vi "Set Scrollbars.vi"(8 "error in (no error)":errorcluster, 10 "Scrollbars":bool, 11 "2DArrayManager in":refnum<class "2DArrayManager.lvclass">) -> (0 "error out":errorcluster, 3 "2DArrayManager out":refnum<class "2DArrayManager.lvclass">)   [LabVIEW 2020, in "OOPanel.lvlib" / "2DArrayManager.lvclass"]
uses:
  2DArrayManager.lvclass
  2DArrayManager.lvclass/2DArrayManager.ctl
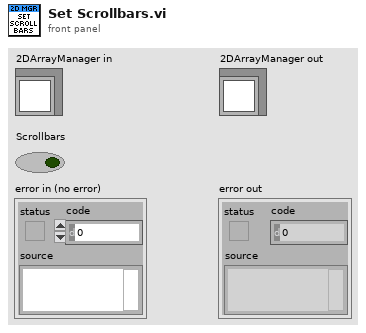
[diagram p1: front panel]
types:
  T1 = typedef "OOPanel.lvlib/2DArrayManager.lvclass/Options.ctl" = cluster{"Running":bool, "Borders":bool, "Background":u32, "V Scroll":bool, "H Scroll":bool, "Blank":refnum<class "2DPanelBlank.lvclass">}
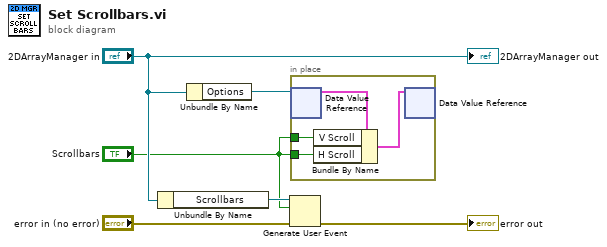
[diagram p0: block diagram]
diagram:
  n1 = Unbundle By Name("2DArrayManager in") -> ("Scrollbars"=w6:refnum<user-event>)
  n2 = Unbundle By Name("2DArrayManager in") -> ("Options"=w3:refnum<data-value>)
  n3 = Generate User Event(user event=w6, event data cluster="Scrollbars", error in="error in (no error)") -> (error out=→"error out":errorcluster)  [unwired: 1 in, 1 out]
  n4 = in-place {
    in-place-border: "Scrollbars" -> [w8]
    in-place-border: "Scrollbars" -> [w7]
    n5 = in-place-dvr #1(w3) -> (w10:T1)  [unwired: 1 out]
    n6 = Bundle By Name(cluster=w10, "V Scroll"=w8, "H Scroll"=w7) -> (w9:T1)
    n7 = in-place-dvr #1(w9) -> ()  [unwired: 2 out]
  }
  "2DArrayManager out" <- "2DArrayManager in"
